vi "InitializeInstrument.vi"(8 "error in (no error)":errorcluster, 11 "reference in":refnum<class "sim_MmW.lvclass">) -> (0 "error out":errorcluster, 3 "reference out":refnum<class "sim_MmW.lvclass">)   [LabVIEW 2019, in "sim_MmW.lvclass"]
doc: "Opens instrument session(s) and performs initial configuration for selected mode.\n\nInputs:\n<b>Initialization source</b> ini file and ini section to be read\n<b>Mode</b> specifies operation mode: BB/IF/RF"
uses:
  sim_MmW.lvclass
  C:/Barkhausen mmWave radar/Development/modules/mmw_instrument/src_LabVIEW/Host/SubVIs/mmWave instrument_class/mmWave instrument.lvclass
  mmWave instrument_class/Instrument state.ctl
  Low-level/TypeDefs/Detected mmWave Adapters.ctl
  <vilib>/userdefined/High Color/nirio_resource_hc.ctl
  Low-level/TypeDefs/mmWave Adapter Information.ctl
  Low-level/TypeDefs/Constants.ctl
  Low-level/Utility/Global Constants.vi
  mmWave instrument_class/mmWave instrument.lvclass
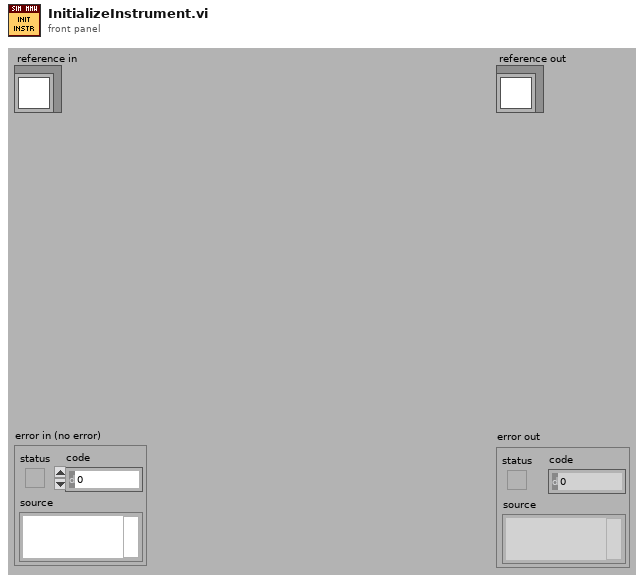
[diagram p1: front panel]
types:
  T1 = typedef "Constants.ctl" = cluster{"data clock rate (Hz)":dbl, "sample rate (Hz)":dbl, "sample rate selector string":string, "default tx bitfile path":path, "default rx bitfile path":path, "default proc bitfile path":path}
  T2 = typedef "mmWave instrument.lvclass/Instrument state.ctl" = enum16{"Off", "Initialization", "Configuration", "Running", "Calibration"}
  T3 = typedef "mmWave instrument.lvclass/ObjectAttributesRef.ctl" = refnum<data-value>
  T4 = typedef "sim_MmW.lvclass/ObjectAttributesRef.ctl" = refnum<data-value>
  T5 = typedef "sim_MmW.lvclass/ObjectAttributes.ctl" = cluster{"RF config":T6, "RX samples":i32, "Downloaded Bursts":map{string, refnum<class "mmWave data.lvclass">}, "TX Fs":dbl, "RX Fs":dbl, "burst sequence":string[], "Burst mode":T7}
  T6 = typedef "mmWave HW Control.lvlib/HW TXRX RF config cluster.ctl" = cluster{"TX.Frequency":dbl, "TX.Gain":dbl, "TX.mmWave adapter":string, "RX.Frequency":dbl, "RX.Gain":dbl, "RX.mmWave adapter":string}
  T7 = typedef "mmWave instrument.lvclass/BurstMode.ctl" = enum16{"burst", "continuous"}
  T8 = typedef "mmWave instrument.lvclass/ObjectAttributes.ctl" = cluster{"mode":T9, "instr state":T2, "Max Fs":dbl, "Equalization coeff":cdb[], "LO sync en":bool, "Trig sync en":bool, "LO sources":T10, "LO Export":T11, "Fc.range":cluster{"min":dbl, "max":dbl}, "Sync mode":T12, "equalization en":bool, "sequence":string[]}
  T9 = typedef "mmWave instrument.lvclass/Instrument mode.ctl" = enum16{"RF", "IF", "BB"}
  T10 = typedef "mmWave HW Control.lvlib/LO sources.ctl" = cluster{"RX/LO1 src":string, "TX/LO1 src":string, "LO2 src":string}
  T11 = typedef "mmWave HW Control.lvlib/LO export.ctl" = cluster{"TX LO1 export":bool, "TX LO1 export level":dbl, "RX LO1 export":bool, "RX LO1 export level":dbl, "LO2 export":bool, "LO2 export level":dbl}
  T12 = typedef "mmWave instrument.lvclass/Sync mode.ctl" = enum16{"Slave", "Master"}
  T13 = typedef "Detected mmWave Adapters.ctl" = cluster{"3620 resource name":T14, "detected mmWave adapters":T15[]}
  T14 = typedef "nirio_resource_hc.ctl" = tag
  T15 = typedef "mmWave Adapter Information.ctl" = cluster{"scope":string, "mmWave adapter type":string, "serial number":u64}
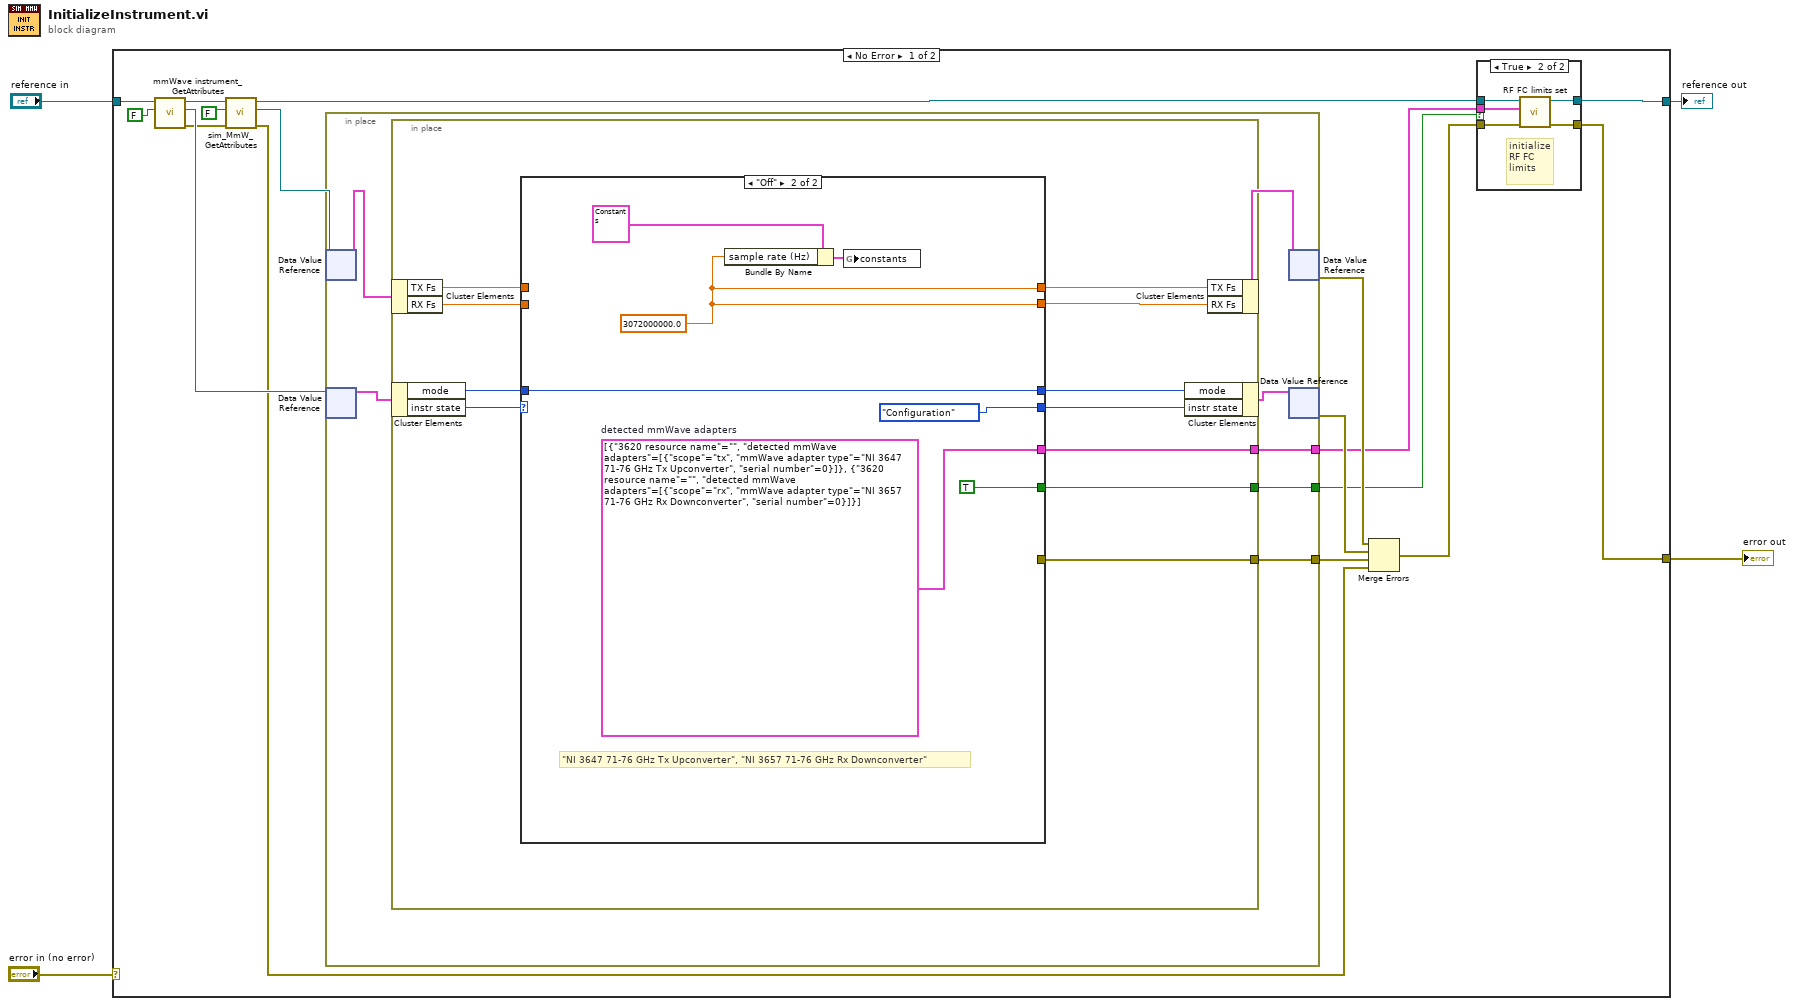
[diagram p0: block diagram]
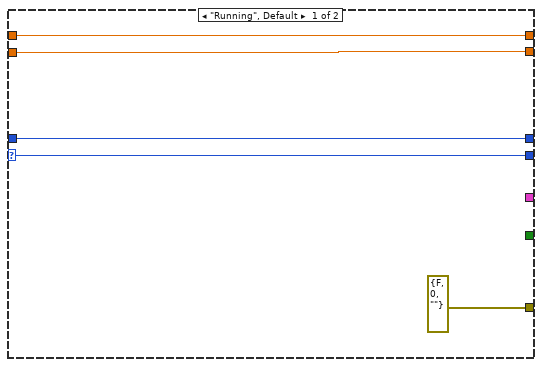
[diagram p3: hidden frame]
diagram:
  n1 = case shown="No Error" "error in (no error)" {
    selector: "error in (no error)" -> [_ w60]
    tunnel: [w6 w60] -> w3
    tunnel: [w9 w59] -> w1
    tunnel: "reference in" -> [w20 w59]
    frame No Error {
      n2 = call "mmWave instrument_GetAttributes.vi"("return data? (T)"=FALSE, "reference in"=w20) -> ("error out"=w13:errorcluster, "attributes ref"=w15:T3, "reference out"=w19:refnum<class "sim_MmW.lvclass">)  [unwired: 6 in, 1 out]
      n3 = call "sim_MmW_GetAttributes.vi"("error in (no error)"=w13, "return data? (T)"=FALSE, "reference in"=w19) -> ("error out"=w10:errorcluster, "attributes ref"=w16:T4, "reference out"=w21:refnum<class "sim_MmW.lvclass">)  [unwired: 5 in, 1 out]
      n4 = in-place {
        in-place-border: [w31] -> w14
        in-place-border: [w30] -> w8
        in-place-border: [w29] -> w5
        n5 = in-place-dvr #1(w16) -> (w35:T5)  [unwired: 1 out]
        n6 = in-place-dvr #2(w15) -> (w33:T8)  [unwired: 1 out]
        n7 = in-place {
          in-place-border: [w45] -> w31
          in-place-border: [w37] -> w30
          in-place-border: [w36] -> w29
          n8 = in-place-cluster #3(w35) -> ("TX Fs"=w39:dbl, "RX Fs"=w38:dbl)
          n9 = in-place-cluster #4(w33) -> ("mode"=w46:T9, "instr state"=w43:T2)
          n10 = case shown="\"Off\"" w43 {
            selector: w43 -> [w47 _]
            tunnel: w46 -> [w51 w58]
            tunnel: [errorcluster {"status"=FALSE, "code"=0, "source"=""} ("error out") _] -> w45
            tunnel: [w47 Instrument_state."Configuration" ("instr state")] -> w44
            tunnel: [w51 w58] -> w42
            tunnel: [w49 w53] -> w41
            tunnel: [w48 w53] -> w40
            tunnel: w39 -> [w49 _]
            tunnel: w38 -> [w48 _]
            tunnel: [_ w55] -> w37
            tunnel: [_ TRUE] -> w36
            frame "Running", Default {
            }
            frame "Off" {
              w53 = 3072000000.0 ("sample rate (Hz)")
              w55 = T13[] [{"3620 resource name"="", "detected mmWave adapters"=[{"scope"="tx", "mmWave adapter type"="NI 3647 71-76 GHz Tx Upconverter", "serial number"=0}]}, {"3620 resource name"="", "detected mmWave adapters"=[{"scope"="rx", "mmWave adapter type"="NI 3657 71-76 GHz Rx Downconverter", "serial number"=0}]}]  # detected mmWave adapters
              # "\"NI 3647 71-76 GHz Tx Upconverter\", \"NI 3657 71-76 GHz Rx Downconverter\""
              n11 = Bundle By Name(cluster=T1 {"data clock rate (Hz)"=0.0, "sample rate (Hz)"=0.0, "sample rate selector string"="", "default tx bitfile path"=path "", "default rx bitfile path"=path "", "default proc bitfile path"=path ""} ("constants"), "sample rate (Hz)"=w53) -> (w52:T1)
              n12 = global write "Global Constants.vi" "constants"(w52) -> ()
            }
          }
          n13 = in-place-cluster #4("mode"=w42, "instr state"=w44) -> (w32:T8)
          n14 = in-place-cluster #3("TX Fs"=w41, "RX Fs"=w40) -> (w34:T5)
        }
        n15 = in-place-dvr #1(w34) -> (w12:errorcluster)  [unwired: 1 out]
        n16 = in-place-dvr #2(w32) -> (w11:errorcluster)  [unwired: 1 out]
      }
      n17 = Merge Errors(w12, w11, w14, w10) -> (w7:errorcluster)
      n18 = case shown="True" w5 {
        tunnel: w21 -> [w23 w28]
        tunnel: [w23 w27] -> w9
        tunnel: w8 -> [_ w26]
        tunnel: w7 -> [w22 w25]
        tunnel: [w22 w24] -> w6
        frame False {
        }
        frame True {
          # "initialize\nRF FC \nlimits"
          n19 = call-dynamic "RF FC limits set.vi"("error in (no error)"=w25, "detected mmWave adapters"=w26, "reference in"=w28) -> ("error out"=w24:errorcluster, "reference out"=w27:refnum<class "sim_MmW.lvclass">)  [unwired: 7 in]
        }
      }
    }
    frame Error {
    }
  }
  "error out" <- w3
  "reference out" <- w1
